vi "index.vi"() -> ()   [LabVIEW 2025]
uses:
  <vilib>/Analysis/3filter.llb/Filter Passband Type.ctl
  <vilib>/Analysis/NI_AALBase.lvlib
panel:
  in  "clearFilterSignalButton":bool
  in  "Vlastnosti filtru":T2={"Typ filtru"=enum."Lowpass", "Filtr"=FALSE, "Horní mezní frekvence"=51.0, "Dolní mezní frekvence\n(mezní frekvence při použití HP, DP)"=49.0}
  in  "název souboru":string
  out "Graf pro porovnání signálu":waveform(dbl)[](graph)
  out "Graf pro porovnání spekter":cluster{"f0":dbl, "df":dbl, "magnitude":dbl[]}[](graph)
  in  "filterSignalButton":bool
  in  "saveSignal":bool
  out "iterace":i32
  out "infoLabel":string
  in  "stop":bool
  in  "loadSignalButton":bool
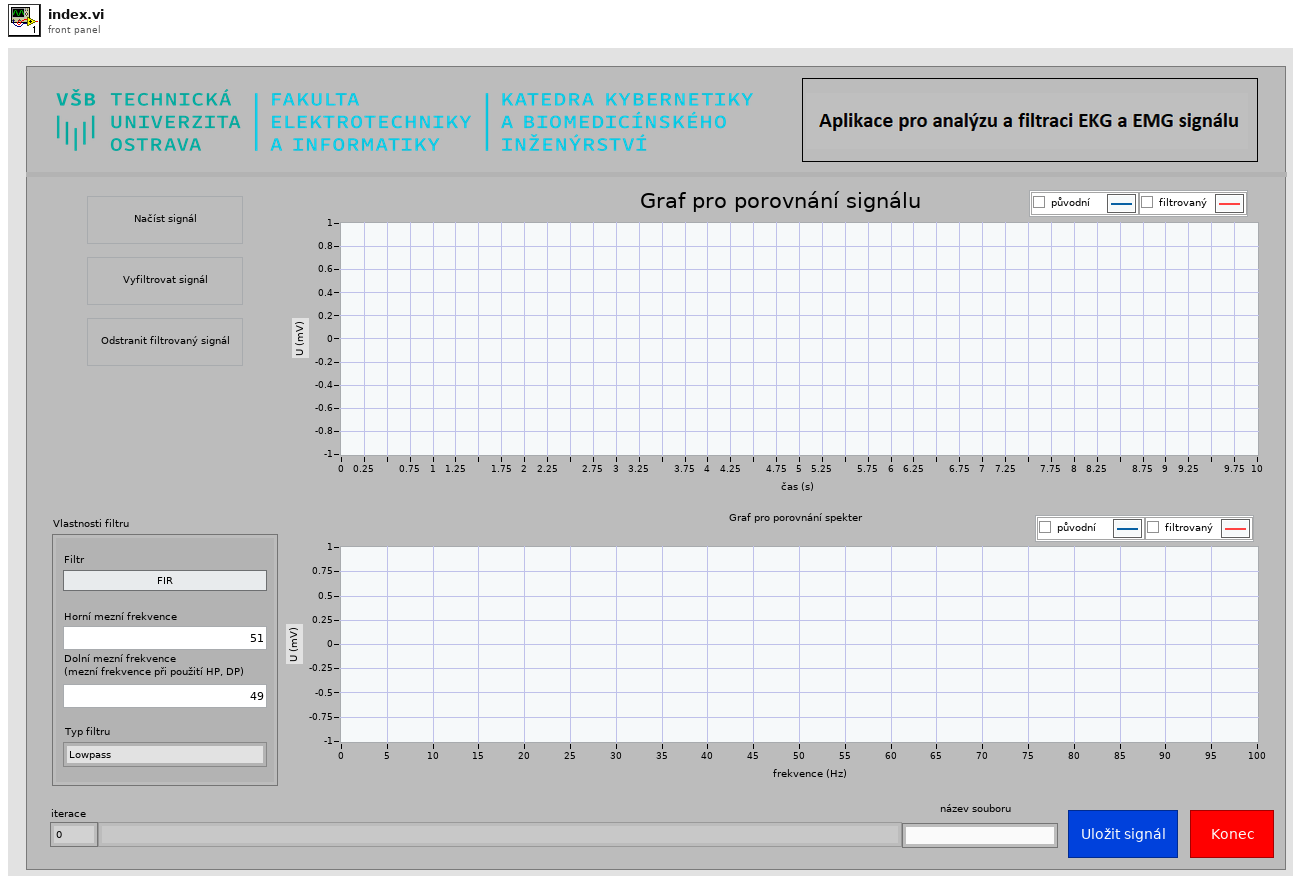
[diagram p1: front panel]
types:
  T1 = typedef "NI_AALBase.lvlib/Filter Passband Type.ctl" = enum32{"Lowpass", "Highpass", "Bandpass", "Bandstop"}
  T2 = cluster{"Typ filtru":T1, "Filtr":bool, "Horní mezní frekvence":dbl, "Dolní mezní frekvence\n(mezní frekvence při použití HP, DP)":dbl}
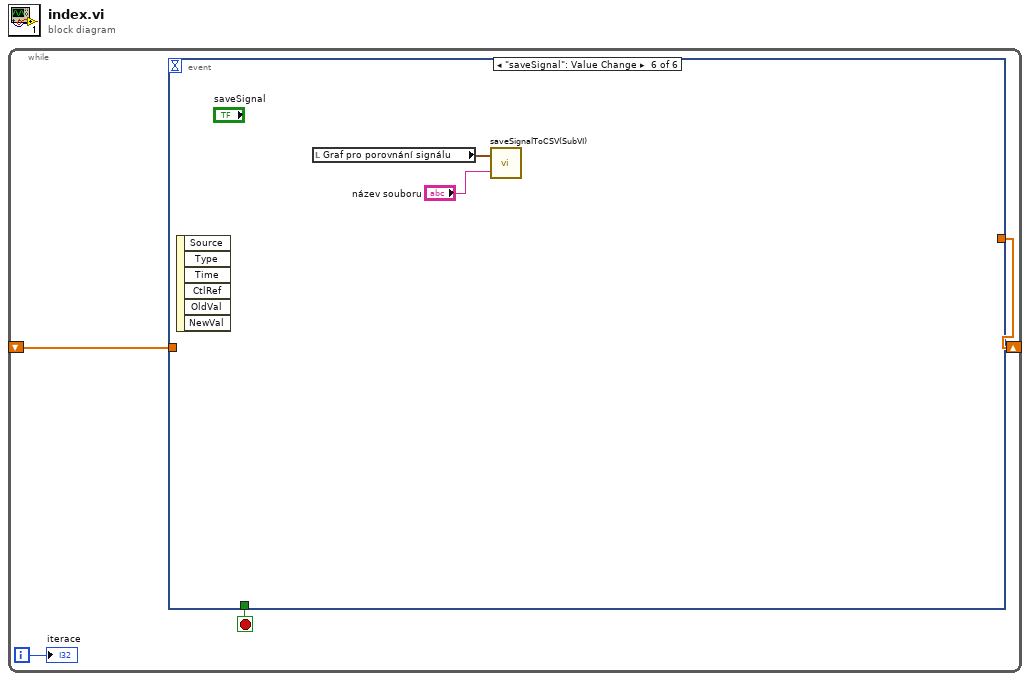
[diagram p0: block diagram]
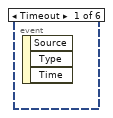
[diagram p2: hidden frame]
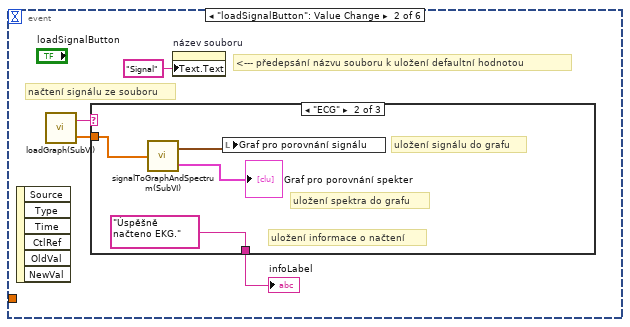
[diagram p3: hidden frame]
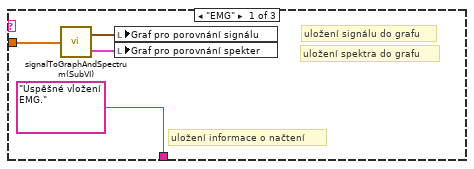
[diagram p4: hidden frame]
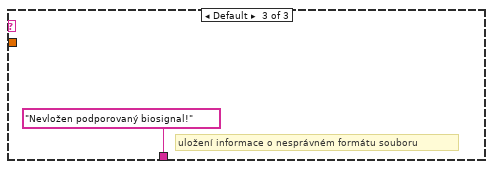
[diagram p5: hidden frame]
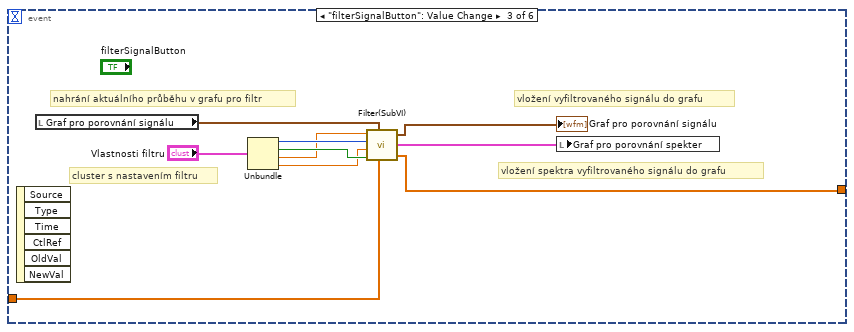
[diagram p6: hidden frame]
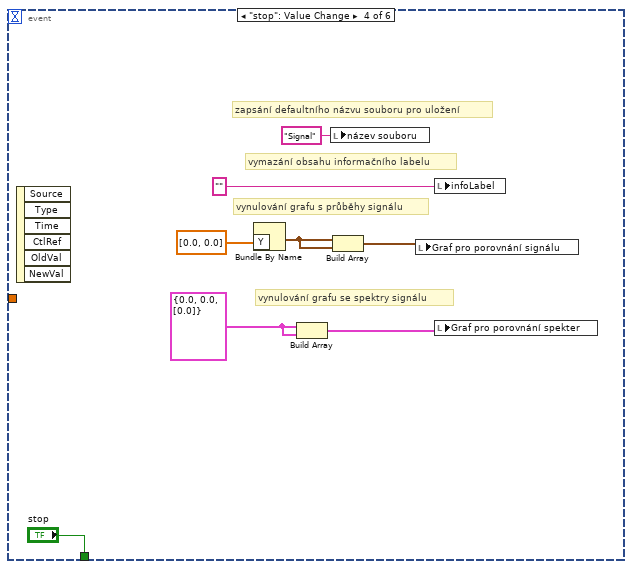
[diagram p7: hidden frame]
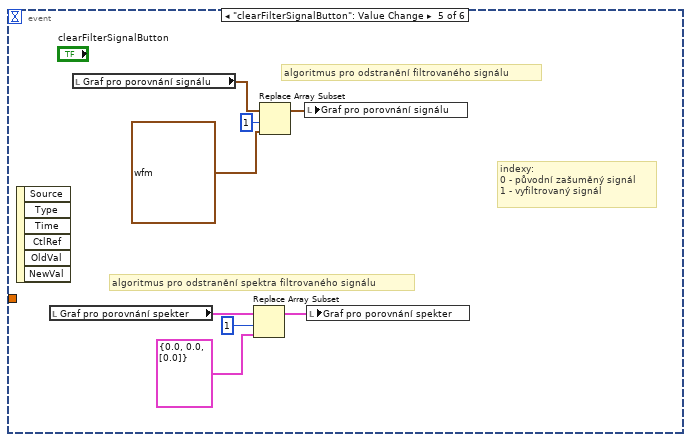
[diagram p8: hidden frame]
diagram:
  n1 = while {
    shift-right: [w2] -> _
    shift-left: _ -> [w1]
    i -> [w3]
    stop <- w4 stop-if-true
    n2 = event shown="[5] \"saveSignal\": Value Change" {
      selector: _ -> [_ _ _ _ _ _]
      dyn-events: _ -> [_ _ _ _ _ _]
      timeout: _ -> [_ _ _ _ _ _]
      tunnel: [_ _ _ "stop" _ _] -> w4
      tunnel: [_ _ w25 _ _ _] -> w2
      tunnel: w1 -> [_ _ w24 _ _ _]
      event Timeout {
        n3 = event-data() -> ()  [unwired: 1 in, 3 out]
      }
      event "loadSignalButton": Value Change {
        # "<--- předepsání názvu souboru k uložení defaultní hodnotou"
        # "načtení signálu ze souboru"
        n4 = event-data() -> ()  [unwired: 1 in, 6 out]
        n5 = call "loadGraph(SubVI).vi"() -> ("String"=w7:string, "Array"=w6:dbl[])  [unwired: 1 in]
        n6 = case shown="\"ECG\"" w7 {
          tunnel: w6 -> [w10 w15 _]
          tunnel: ["Úspěšné vložení EMG." ("String") "Úspěšně načteno EKG." ("String") "Nevložen podporovaný biosignal!"] -> w8
          frame "EMG" {
            # "uložení spektra do grafu"
            # "uložení signálu do grafu"
            # "uložení informace o načtení"
            n7 = call "signalToGraphAndSpectrum(SubVI).vi"("Vstupní signál"=w10) -> ("Signál do grafu"=w12:waveform(dbl)[], "Spektrum do grafu"=w11:cluster{"f0":dbl, "df":dbl, "magnitude":dbl[]}[])
            n8 = local write "Graf pro porovnání signálu"(w12) -> ()
            n9 = local write "Graf pro porovnání spekter"(w11) -> ()
          }
          frame "ECG" {
            # "uložení spektra do grafu"
            # "uložení signálu do grafu"
            # "uložení informace o načtení"
            n10 = call "signalToGraphAndSpectrum(SubVI).vi"("Vstupní signál"=w15) -> ("Signál do grafu"=w13:waveform(dbl)[], "Spektrum do grafu"=→"Graf pro porovnání spekter":cluster{"f0":dbl, "df":dbl, "magnitude":dbl[]}[])
            n11 = local write "Graf pro porovnání signálu"(w13) -> ()
          }
          frame Default {
            # "uložení informace o nesprávném formátu souboru"
          }
        }
        "infoLabel" <- w8
        n12 = property on="název souboru" class="Str"("Text.Text"="Signal") -> ()  [unwired: 2 in, 2 out]
      }
      event "filterSignalButton": Value Change {
        # "vložení spektra vyfiltrovaného signálu do grafu"
        # "vložení vyfiltrovaného signálu do grafu"
        # "nahrání aktuálního průběhu v grafu pro filtr"
        # "cluster s nastavením filtru"
        n13 = event-data() -> ()  [unwired: 1 in, 6 out]
        n14 = local read "Graf pro porovnání signálu"() -> (w23:waveform(dbl)[])
        n15 = Unbundle("Vlastnosti filtru") -> ("Typ filtru"=w21:T1, "Filtr"=w20:bool, "Horní mezní frekvence"=w19:dbl, "Dolní mezní frekvence\n(mezní frekvence při použití HP, DP)"=w18:dbl)
        n16 = call "Filter(SubVI).vi"("Horní mezní frekvence"=w19, "Vstupní signál"=w23, "Druh filtru"=w21, "Dolní mezní frekvence"=w18, "Vstup z registru"=w24, "Typ filtru"=w20) -> ("Signál"=→"Graf pro porovnání signálu":waveform(dbl)[], "Spektrum"=w26:cluster{"f0":dbl, "df":dbl, "magnitude":dbl[]}[], "Výstup filtrovaného signálu"=w25:dbl[])
        n17 = local write "Graf pro porovnání spekter"(w26) -> ()
      }
      event "stop": Value Change {
        w30 = cluster{"f0":dbl, "df":dbl, "magnitude":dbl[]} {"f0"=0.0, "df"=0.0, "magnitude"=[0.0]} ("Spektrum")
        # "vynulování grafu se spektry signálu"
        # "vynulování grafu s průběhy signálu"
        # "vymazání obsahu informačního labelu"
        # "zapsání defaultního názvu souboru pro uložení"
        n18 = event-data() -> ()  [unwired: 1 in, 6 out]
        n19 = Bundle By Name("Y"=dbl[] [0.0, 0.0]) -> (w31:waveform(dbl))  [unwired: 1 in]
        n20 = Build Array(w30, w30) -> (w29:cluster{"f0":dbl, "df":dbl, "magnitude":dbl[]}[])
        n21 = local write "název souboru"("Signal" ("název souboru")) -> ()
        n22 = Build Array(w31, w31) -> (w32:waveform(dbl)[])
        n23 = local write "Graf pro porovnání signálu"(w32) -> ()
        n24 = local write "infoLabel"("" ("String")) -> ()
        n25 = local write "Graf pro porovnání spekter"(w29) -> ()
      }
      event "clearFilterSignalButton": Value Change {
        # "indexy:\n0 - původní zašuměný signál\n1 - vyfiltrovaný signál"
        # "algoritmus pro odstranění spektra filtrovaného signálu"
        # "algoritmus pro odstranění filtrovaného signálu"
        n26 = event-data() -> ()  [unwired: 1 in, 6 out]
        n27 = local read "Graf pro porovnání spekter"() -> (w37:cluster{"f0":dbl, "df":dbl, "magnitude":dbl[]}[])
        n28 = local read "Graf pro porovnání signálu"() -> (w43:waveform(dbl)[])
        n29 = Replace Array Subset(array=w37, new element=cluster{"f0":dbl, "df":dbl, "magnitude":dbl[]} {"f0"=0.0, "df"=0.0, "magnitude"=[0.0]} ("new element/subarray"), index=1) -> (w38:cluster{"f0":dbl, "df":dbl, "magnitude":dbl[]}[])
        n30 = Replace Array Subset(array=w43, new element=waveform(dbl) {"t0"=timestamp(0 s since 1904-01-01), "dt"=0.0, "Y"=[0.0]} ("new element/subarray"), index=1) -> (w40:waveform(dbl)[])
        n31 = local write "Graf pro porovnání signálu"(w40) -> ()
        n32 = local write "Graf pro porovnání spekter"(w38) -> ()
      }
      event "saveSignal": Value Change {
        n33 = event-data() -> ()  [unwired: 1 in, 6 out]
        n34 = local read "Graf pro porovnání signálu"() -> (w44:waveform(dbl)[])
        n35 = call "saveSignalToCSV(SubVI).vi"("název souboru"="název souboru", "Graf pro porovnání signálu"=w44) -> ()  [unwired: 1 in]
      }
    }
    "iterace" <- w3
  }
